vi "Save_interim_img.vi"() -> ()   [LabVIEW 2020]
uses:
  <vilib>/Utility/file.llb/Write Delimited Spreadsheet (I64).vi
panel:
  out "Elapsed time [ms]":u32
  in  "h":i32=10 min=1 max=5000 step=1
  in  "w":i32=1 min=1 max=5000 step=1
  out "error out":errorcluster
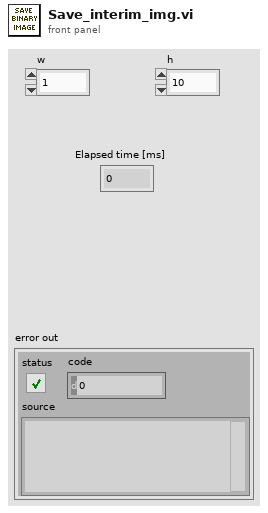
[diagram p1: front panel]
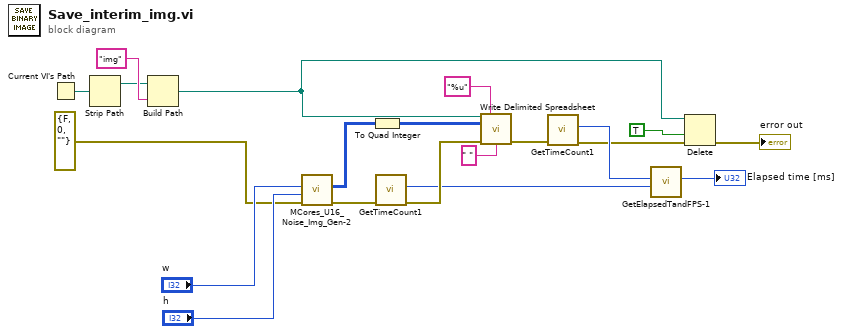
[diagram p0: block diagram]
diagram:
  n1 = Current VI's Path() -> (path=w20:path)
  n2 = Strip Path(path=w20) -> (stripped path=w18:path)  [unwired: 1 out]
  n3 = Build Path(base path=w18, name or relative path="img" ("string")) -> (appended path=w2:path)
  n4 = call "MCores_U16_Noise_Img_Gen-2.vi"("error IN"=errorcluster {"status"=FALSE, "code"=0, "source"=""} ("error in (no error)"), "[IN] Width"="h", "[IN] Height"="w") -> ("error OUT"=w10:errorcluster, "[OUT] U16 Pixel Img"=w13:u16[][])  [unwired: 7 in]
  n5 = To Quad Integer(1:w13) -> (0:w12:i64[][])
  n6 = call "GetTimeCount1.vi"("error IN"=w10) -> ("error OUT"=w9:errorcluster, "[OUT] Timer Count"=w6:u32)  [unwired: 9 in]
  n7 = call-poly <vilib>:"Write Delimited Spreadsheet.vi"("file path (dialog if empty)"=w2, "format (%d)"="%u", "2D data"=w12, "error in (no error)"=w9, "delimiter (\\t)"=" " ("delimiter (\\t)")) -> ("error out"=w8:errorcluster)  [unwired: 9 in, 1 out]
  n8 = call "GetTimeCount1.vi"("error IN"=w8) -> ("error OUT"=w4:errorcluster, "[OUT] Timer Count"=w7:u32)  [unwired: 9 in]
  n9 = call "GetElapsedTandFPS-1.vi"("[IN] Timer Count Before ALL [ms]"=w6, "[IN] Timer Count After ALL [ms]"=w7) -> ("[OUT] Elapsed time [ms]"=→"Elapsed time [ms]":u32)  [unwired: 3 in, 2 out]
  n10 = Delete(path (use dialog)=w2, confirm (F)=TRUE, error in=w4) -> (error out=→"error out":errorcluster)  [unwired: 2 in, 2 out]
